vi "NewProjectDialog.vi"(10 "Project XML":string="<ProjectTemplate>\n  <Title localize=\"yes\">队列状态机</Title>\n  <Description localize=\"yes\">本模板可用于创建事件驱动的用户界面状态机。</Description>\n  <Filter localize=\"yes\">桌面：模板</Filter>\n  <Keywords localize=\"yes\">状态;状态机;队列;事件;处理器;消息</Keywords>\n  <LocationPath>Core/Queued State Machine</LocationPath>\n  <ProjectPath>Queued State Machine.lvproj</ProjectPath>\n  <ListboxImagePath>images/qsm_small.png</ListboxImagePath>\n  <GalleryImagePaths>images/qsm.png;images/knob.jpg</GalleryImagePaths>\n  <DocumentationPath>html/Project Documentation.html</DocumentationPath>\n  <CustomVIMode>None</CustomVIMode>\n  <CustomVIPath></CustomVIPath>\n</ProjectTemplate>" caption="项目XML", 11 "Calling Mode":T1 caption="调用模式") -> ()   [LabVIEW 2016]
uses:
  <resource>/dialog/NewProjectWizard/NewProjectDialogCallingModes.ctl
  <resource>/dialog/NewProjectWizard/MetaDataObj/MetaDataObj.lvclass
  <resource>/dialog/NewProjectWizard/SpecPage/Base/BaseSpecPage.lvclass
  <resource>/dialog/NewProjectWizard/Operation to Log.ctl
  <vilib>/event_ctls.llb/eventvkey.ctl
  <resource>/dialog/NewProjectWizard/MetaDataObj/MetaDataObj.lvclass/MetaDataObj.ctl
  <resource>/dialog/NewProjectWizard/Spec Page Interface.ctl
  <resource>/dialog/NewProjectWizard/MetaDataObj/Accessors/Write Project Root.vi
  <resource>/dialog/NewProjectWizard/MetaDataObj/Accessors/Read Project Root.vi
  <resource>/dialog/NewProjectWizard/MetaDataObj/Accessors/Read File Prefix.vi
  <resource>/dialog/NewProjectWizard/MetaDataObj/Accessors/Read Project Name.vi
  <resource>/dialog/NewProjectWizard/MetaDataObj/Accessors/Read Overlay Pixmap.vi
  <resource>/dialog/NewProjectWizard/MetaDataObj/Accessors/Read Custom VI Mode.vi
  <resource>/dialog/NewProjectWizard/MetaDataObj/Accessors/Read Custom VI Path.vi
  <resource>/dialog/NewProjectWizard/MetaDataObj/Accessors/Read Title.vi
  <resource>/dialog/NewProjectWizard/MetaDataObj/Accessors/Read Project Path.vi
  <vilib>/LabVIEW Icon API/lv_icon/Classes/Icon/Icon.lvclass
  <helpdir>/_LaunchHelp.vi
  <resource>/dialog/NewProjectWizard/Init Search Page.vi
  <resource>/dialog/NewProjectWizard/Build Error String.vi
  <resource>/dialog/NewProjectWizard/Log Project Selection.vi
  <resource>/dialog/NewProjectWizard/Process Tab Key.vi
  <resource>/dialog/lvconfig.llb/LV Config Read Pathlist.vi
  <resource>/dialog/NewProjectWizard/MetaDataObj/Convert To Child Class.vi
  <resource>/dialog/NewProjectWizard/Init Spec Page.vi
  <resource>/dialog/NewProjectWizard/Defer Panel Updates.vi
  <resource>/dialog/NewProjectWizard/ValidateFilePath.vi
  <resource>/dialog/lvconfig.llb/LV Config Write Pathlist.vi
  <resource>/dialog/NewProjectWizard/Project Copying/CreateUserProject.vi
  <resource>/dialog/NewProjectWizard/Project Copying/NI_NPW_Project Copying.lvlib
  <vilib>/Utility/cursorutil.llb/Set Busy.vi
  <resource>/dialog/NewProjectWizard/Project Copying/SaveTemplatePathToINI.vi
  <resource>/dialog/NewProjectWizard/FindRecentItem.vi
  <resource>/dialog/NewProjectWizard/Loading Project Info/LoadTemplateFromXML.vi
  <resource>/dialog/NewProjectWizard/Loading Project Info/NI_NPW_Loading Project Info.lvlib
panel:
  in  "Dummy Template":refnum<class "MetaDataObj.lvclass"> caption="虚设模板"
  in  "recent_item":path caption="最近项"
  out "Title":string="消息:" caption="标题"
  in  "Spec Page Title":string="配置新项目：%s" caption="规范页标题"
  in  "Search Page Title":string="选择项目起始位置：" caption="搜索页标题"
  out "Error Messages":string caption="错误信息"
  out "CurPage Ctrl #n":refnum<vi> caption="当前页Ctrl #n"
  out "CurPage Ctrl #1":refnum<vi> caption="当前页Ctrl #1"
  out "Search Page":refnum<vi> caption="搜索页"
  out "SpecPage Ctrl #n":refnum<vi> caption="规范页Ctrl #n"
  out "SearchPage Ctrl #n":refnum<vi> caption="搜索页Ctrl #n"
  out "SpecPage Ctrl #1":refnum<vi> caption="规范页Ctrl #1"
  out "SearchPage Ctrl #1":refnum<vi> caption="搜索页Ctrl #1"
  in  "Finish":string="完成" caption="完成"
  in  "Next":string="下一步" caption="下一步"
  in  "Help":bool caption="帮助"
  in  "Cancel":bool caption="取消"
  in  "Next":bool caption="下一步"
  in  "Back":bool caption="上一步"
  in  "File Not Found":string="LabVIEW无法找到项目的源文件。" caption="未找到文件"
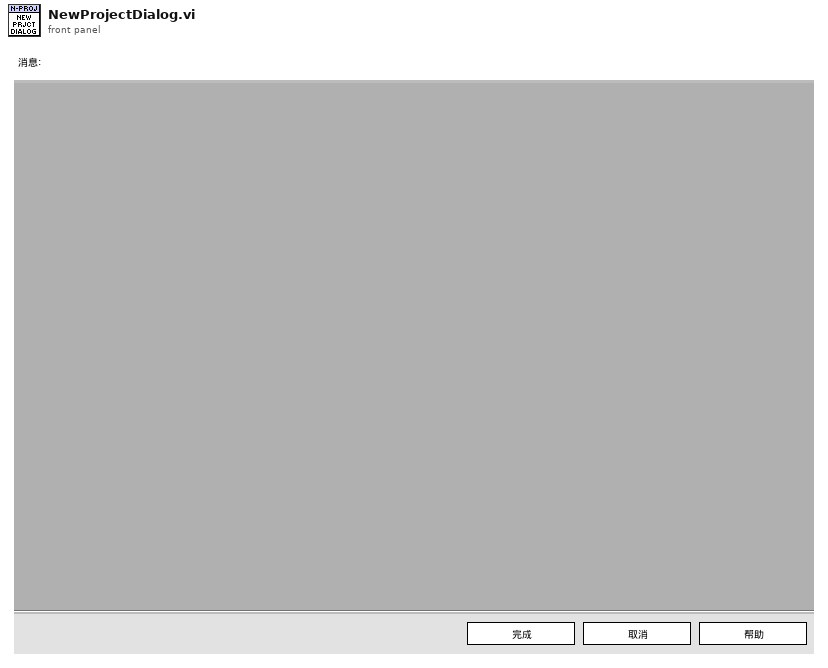
[diagram p1: front panel]
types:
  T1 = typedef "NewProjectDialogCallingModes.ctl" = enum16{"Default", "Open to 2nd Page", "Open Recent Item"}
  T2 = enum32{"Invalid", "Standard", "Closed", "Hidden", "Minimized", "Maximized"}
  T3 = enum8{"Enabled", "Disabled", "Disabled and Grayed Out"}
  T4 = typedef "CustomVIModes.ctl" = enum16{"None", "AfterPage1", "AfterPage2WithUI", "AfterPage2NoUI"}
  T5 = typedef "Operation to Log.ctl" = enum16{"Create", "Cancel", "MoreInfoLink"}
  T6 = typedef "eventvkey.ctl" = enum16{"ASCII", "Enter", "Return", "Shift", "Ctrl", "Alt", "Cmd", "Opt", "Caps", "NumLock", "Clear", "Break", "Up", "Down", "Left", "Right", "Insert", "Delete", "Home", "End", "PageUp", "PageDown", "Escape", "Help", "Pause", "ScrollLock", "F1", "F2", "F3", "F4", "F5", "F6", "F7", "F8", "F9", "F10", "F11", "F12", "F13", "F14", "F15", "F16", "F17", "F18", "F19", "F20", "F21", "F22", "F23", "F24", "Play", "VolumeUp", "VolumeDown", "Mute", "Two Byte Char"}
  T7 = typedef "Spec Page Interface.ctl" = cluster{"\"Tab Forward To\" Refnum":refnum<vi>, "\"Tab Backward To\" Refnum":refnum<vi>, "Errors":refnum<user-event>, "Quit":refnum<user-event>}
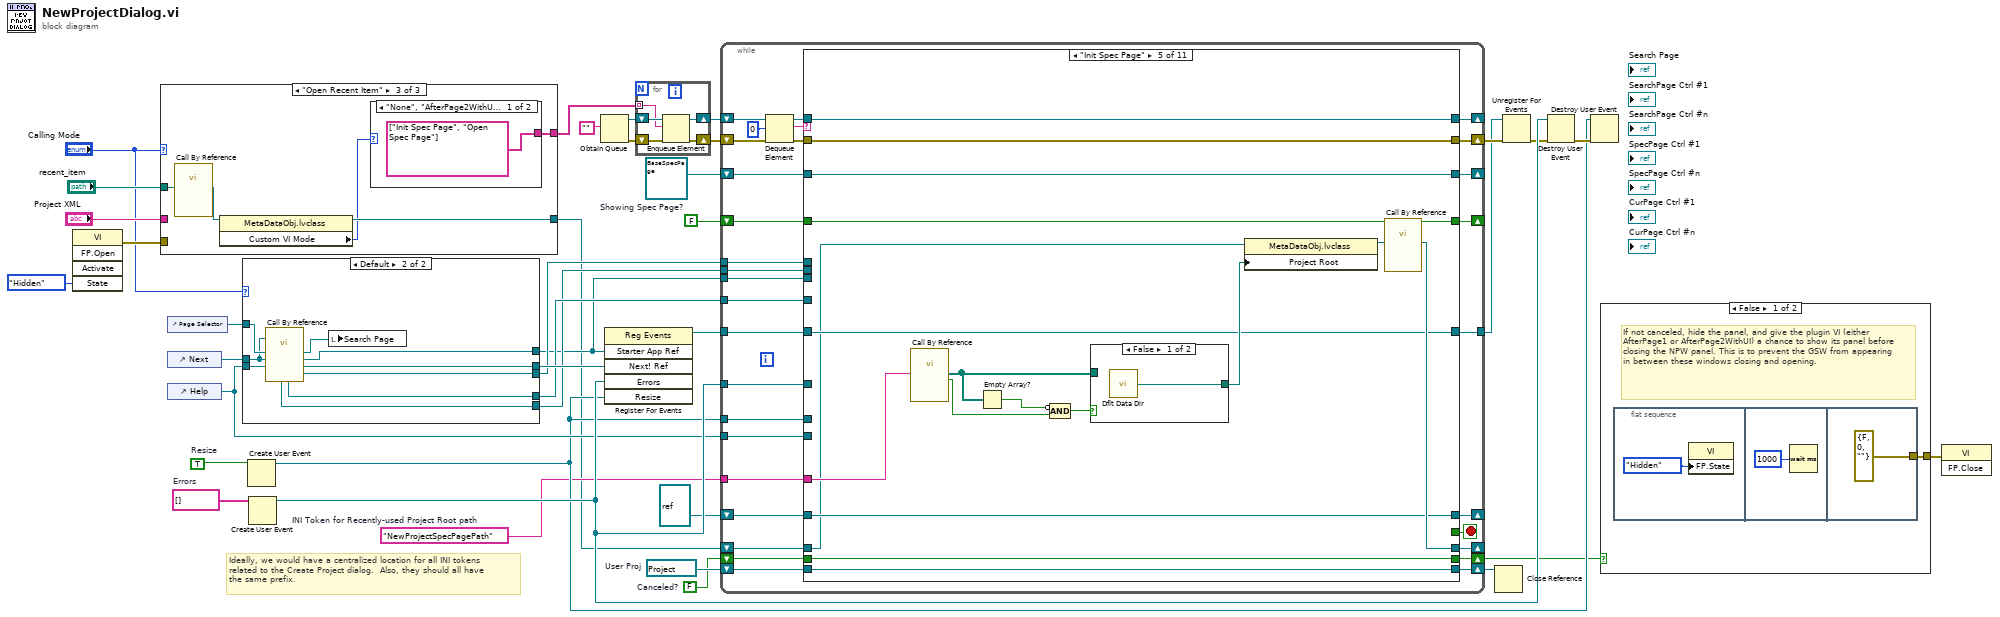
[diagram p0: block diagram]
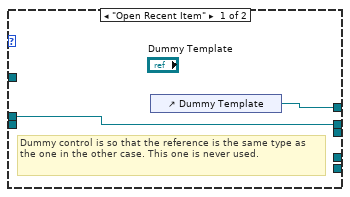
[diagram p3: hidden frame]
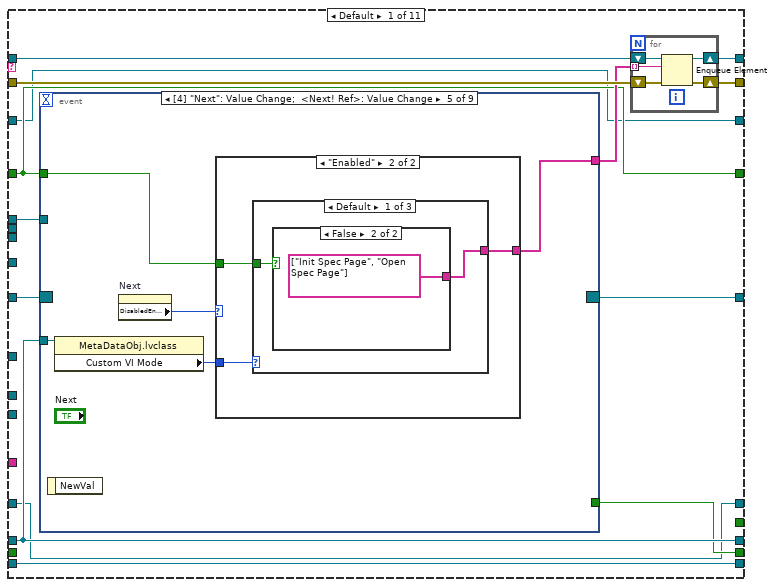
[diagram p4: hidden frame]
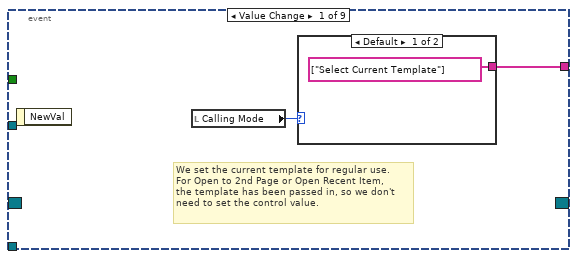
[diagram p5: hidden frame]
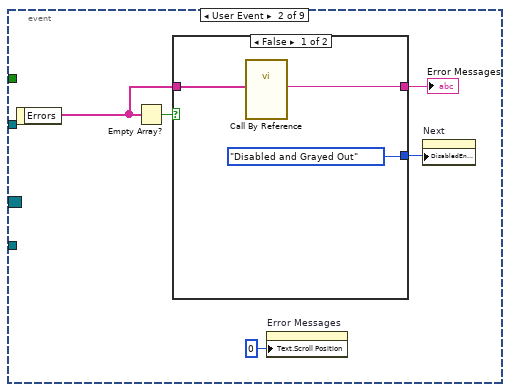
[diagram p7: hidden frame]
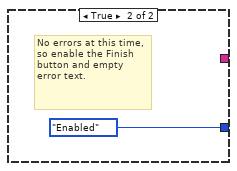
[diagram p8: hidden frame]
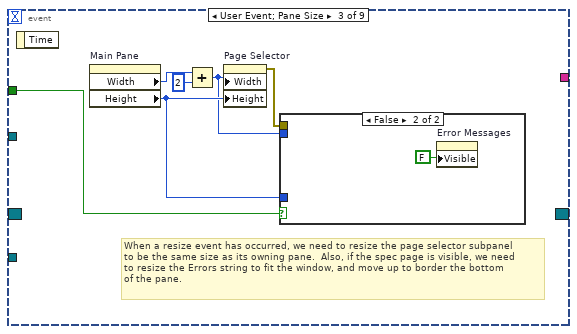
[diagram p9: hidden frame]
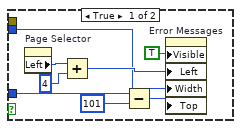
[diagram p10: hidden frame]
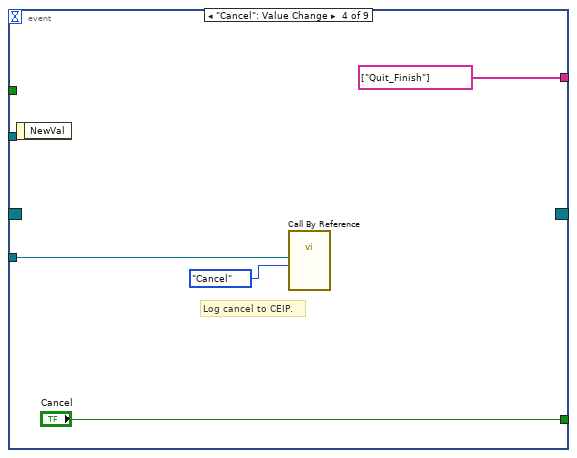
[diagram p11: hidden frame]
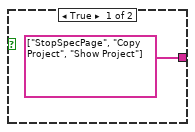
[diagram p13: hidden frame]
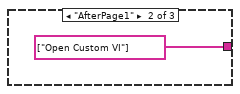
[diagram p14: hidden frame]
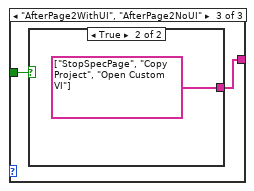
[diagram p15: hidden frame]
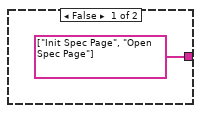
[diagram p16: hidden frame]
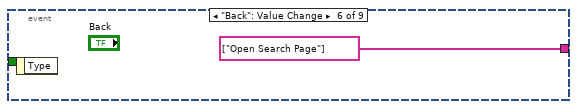
[diagram p17: hidden frame]
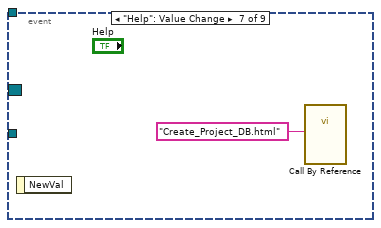
[diagram p18: hidden frame]
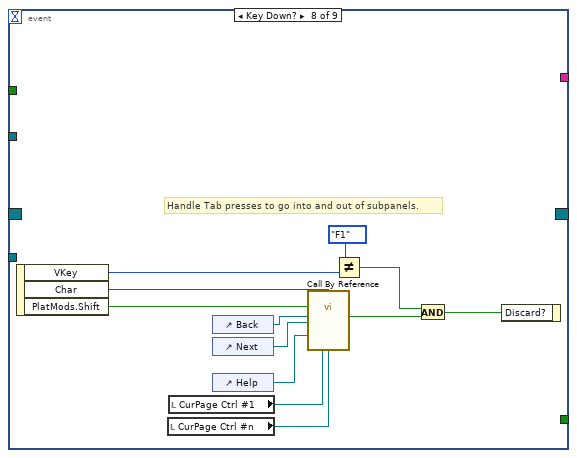
[diagram p19: hidden frame]
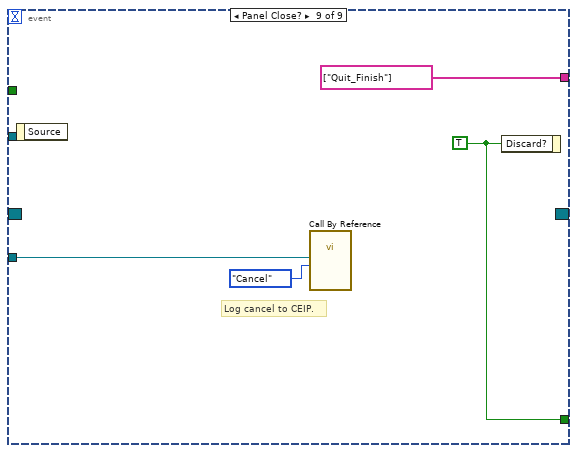
[diagram p20: hidden frame]
diagram:
  w10 = FALSE  # Canceled?
  w12 = "NewProjectSpecPagePath"  # INI Token for Recently-used Project Root path
  w18 = refnum<vi> refnum  # User Proj
  w19 = FALSE  # Showing Spec Page?
  w28 = TRUE  # Resize
  w29 = string[] []  # Errors
  # "Ideally, we would have a centralized location for all INI tokens\nrelated to the Create Project dialog.  Also, they should all have\nthe same prefix."
  n1 = invoke class="VI" method="FP.Open"("State"=T2."Hidden") -> (error out=w17:errorcluster)  [unwired: 4 in, 4 out]
  n2 = case shown="\"Open Recent Item\"" "Calling Mode" {
    tunnel: [string[] ["Select Current Template", "Open Search Page"] ("Initial States") string[] ["Init Spec Page", "Open Spec Page"] ("Initial States") w48] -> w38
    tunnel: "Project XML" -> [_ w41 _]
    tunnel: [_ w40 w47] -> w3
    tunnel: "recent_item" -> [_ _ w45]
    tunnel: w17 -> [_ _ _]
    frame Default {
    }
    frame "Open to 2nd Page" {
      # "(In this mode, the user passes\nin XML for the template that\nthey want.)"
      n3 = call-by-ref "?"("XML String In"=w41) -> ("Template Out"=w40:refnum<class "MetaDataObj.lvclass">)  [unwired: 11 in, 3 out]
      n4 = property on="Back" class="Bool"("DisabledEnum"=T3."Disabled and Grayed Out" ("Disabled")) -> ()  [unwired: 2 in, 2 out]
    }
    frame "Open Recent Item" {
      n5 = call-by-ref "?"("recent_item"=w45) -> ("MetaDataObj out"=w44:refnum<class "MetaDataObj.lvclass">)  [unwired: 11 in, 3 out]
      n6 = property class="MetaDataObj.lvclass"(reference=w44) -> (reference out=w47:refnum<class "MetaDataObj.lvclass">, "Custom VI Mode"=w46:T4)  [unwired: 1 in, 1 out]
      n7 = case shown="\"None\", \"AfterPage2WithUI\", \"AfterPage2NoUI\"" w46 {
        tunnel: [string[] ["Init Spec Page", "Open Spec Page"] ("Initial States") string[] ["Open Custom VI"] ("Initial States")] -> w48
        frame "None", "AfterPage2WithUI", "AfterPage2NoUI" {
        }
        frame "AfterPage1" {
        }
      }
    }
  }
  n8 = control-ref of="Page Selector"() -> (w30:refnum<vi>)
  n9 = control-ref of="Next"() -> (w15:refnum<vi>)
  n10 = control-ref of="Help"() -> (w16:refnum<vi>)
  n11 = case shown="Default" "Calling Mode" {
    tunnel: [w51 w53] -> w7
    tunnel: [w52 w61] -> w37
    tunnel: [_ w60] -> w34
    tunnel: [_ w59] -> w33
    tunnel: w30 -> [_ w57]
    tunnel: w16 -> [_ w56]
    tunnel: w15 -> [w52 w54]
    tunnel: [_ w55] -> w13
    frame "Open Recent Item" {
      # "Dummy control is so that the reference is the same type as the one in the other case. This one is never used."
      n12 = control-ref of="Dummy Template"() -> (w51:refnum<vi>)
    }
    frame Default {
      n13 = call-by-ref "?"("Next Button"=w54, "\"Tab Backward To\" Refnum"=w56, "\"Tab Forward To\" Refnum"=w54, "SubPanel"=w57) -> ("Additional Search Ref"=w55:refnum<vi>, "Next! Ref"=w61:refnum<vi>, "Starter App Ref"=w53:refnum<vi>, "Search Page Ref"=w58:refnum<vi>, "SearchPage Ctrl #n Ref"=w60:refnum<vi>, "SearchPage Ctrl #1 Ref"=w59:refnum<vi>)  [unwired: 4 in, 2 out]
      n14 = local write "Search Page"(w58) -> ()
    }
  }
  n15 = Create User Event(user event datatype=w28) -> (user event=w14:refnum<user-event>)  [unwired: 1 in, 1 out]
  n16 = Create User Event(user event datatype=w29) -> (user event=w35:refnum<user-event>)  [unwired: 1 in, 1 out]
  n17 = Obtain Queue(element data type="") -> (queue out=w23:refnum<queue>, error out=w22:errorcluster)  [unwired: 4 in, 1 out]
  n18 = register-events(w7, w37, w35, w14) -> (reference out=w24:refnum<event-registration>)  [unwired: 2 in, 1 out]
  n19 = for {
    shift-right: [w66] -> w26
    shift-left: w23 -> [w64]
    shift-right: [w65] -> w25
    shift-left: w22 -> [w63]
    tunnel: w38 -> [w62] mode=indexing
    n20 = Enqueue Element(queue=w64, element=w62, error in (no error)=w63) -> (queue out=w66:refnum<queue>, error out=w65:errorcluster)  [unwired: 1 in, 1 out]
  }
  n21 = while {
    shift-right: [w91] -> _
    shift-left: w26 -> [w96]
    shift-right: [w90] -> w21
    shift-left: w25 -> [w95]
    shift-right: [w86] -> _
    shift-left: w3 -> [w87]
    tunnel: w7 -> [w85]
    tunnel: w35 -> [w84]
    tunnel: w34 -> [w83]
    tunnel: w33 -> [w82]
    tunnel: w14 -> [w81]
    shift-right: [w79] -> _
    shift-left: w19 -> [w80]
    shift-right: [w77] -> w11
    shift-left: w18 -> [w78]
    tunnel: w16 -> [w76]
    tunnel: w13 -> [w75]
    tunnel: w12 -> [w74]
    shift-right: [w72] -> w2
    shift-left: w10 -> [w73]
    shift-right: [w71] -> _
    shift-left: refnum<vi> refnum ("vi reference") -> [w70]
    tunnel: w24 -> [w89]
    tunnel: [w69] -> w8
    shift-right: [w68] -> _
    shift-left: refnum<class "BaseSpecPage.lvclass"> refnum ("BaseSpecPage out") -> [w67]
    stop <- w88 stop-if-true
    n22 = Dequeue Element(queue=w96, timeout in ms (-1)=0, error in (no error)=w95) -> (queue out=w94:refnum<queue>, element=w92:string, error out=w93:errorcluster)  [unwired: 1 out]
    n23 = case shown="\"Init Spec Page\"" w92 {
      tunnel: w94 -> [w108 w193 w214 w252 w299 w306 w373 w404 w460 w475 w500]
      tunnel: w93 -> [w109 w192 w210 w249 w298 w305 w378 w405 w459 w473 w499]
      tunnel: [w111 w193 w214 w251 w299 w306 w372 w403 w458 w474 w500] -> w91
      tunnel: [w110 w192 w210 w250 w298 w305 w376 w402 w457 w472 w499] -> w90
      tunnel: w89 -> [w107 w188 w199 w245 w294 w304 w385 w410 w455 w477 w489]
      tunnel: [_ _ _ _ _ _ _ _ _ _ TRUE] -> w88
      tunnel: w87 -> [w105 _ w213 w246 w283 w323 w374 w416 w461 w469 w486]
      tunnel: [w105 w190 w213 w246 w295 w323 w386 w416 w461 w469 w486] -> w86
      tunnel: w85 -> [_ w189 _ _ _ _ _ _ _ _ _]
      tunnel: w84 -> [_ _ _ _ _ w322 _ _ _ _ _]
      tunnel: w83 -> [_ _ w212 _ _ _ _ _ _ _ _]
      tunnel: w82 -> [_ _ w211 _ _ _ _ _ _ _ _]
      tunnel: [w104 w188 w199 w245 w294 w304 w385 w410 w455 w477 w489] -> w69
      tunnel: w81 -> [_ _ w202 _ _ w319 _ _ _ _ _]
      tunnel: w80 -> [w103 w187 _ w244 w293 _ w371 w409 w454 w476 w488]
      tunnel: [w103 w187 w207 w244 w293 w318 w371 w409 w454 w476 w488] -> w79
      tunnel: w78 -> [w102 w186 w205 w242 w288 w317 w384 w408 w453 w470 w487]
      tunnel: [w102 w186 w205 w242 w288 w317 w384 w407 refnum<vi> refnum ("User Proj") w470 w487] -> w77
      tunnel: w76 -> [_ _ _ _ _ w315 _ _ _ _ _]
      tunnel: w75 -> [w101 _ _ _ _ _ _ _ _ _ _]
      tunnel: w74 -> [_ _ _ _ w287 _ _ w406 _ _ _]
      tunnel: w73 -> [_ w185 w198 w241 w286 w312 w383 w401 w450 w467 w485]
      tunnel: [w100 w185 w198 w241 w286 w312 w383 w401 w450 w467 w485] -> w72
      tunnel: [w99 w184 w197 w240 w285 w311 w382 w400 w449 w466 w484] -> w71
      tunnel: w70 -> [w99 w184 w197 w239 w285 w311 w382 w400 w449 w466 w484]
      tunnel: [w98 w183 w196 w238 w284 w310 w381 w399 w448 w465 w478] -> w68
      tunnel: w67 -> [w98 w183 w196 w238 w284 w308 w380 w399 w448 w465 w478]
      frame Default {
        n24 = event shown="[4] \"Next\": Value Change;  <Next! Ref>: Value Change" {
          selector: w107 -> [_ _ _ _ _ _ _ _ _]
          dyn-events: [_ _ _ _ _ _ _ _ _] -> w104
          timeout: _ -> [_ _ _ _ _ _ _ _ _]
          tunnel: [w118 _ _ string[] ["Quit_Finish"] w151 string[] ["Open Search Page"] _ _ string[] ["Quit_Finish"]] -> w106
          tunnel: w105 -> [_ _ _ w146 w150 _ _ _ w181]
          tunnel: w103 -> [_ _ w134 _ w149 _ _ _ _]
          tunnel: w101 -> [_ _ _ _ _ _ _ _ _]
          tunnel: [_ _ _ "Cancel" _ _ _ _ w179] -> w100
          event Value Change {
            # "We set the current template for regular use.\nFor Open to 2nd Page or Open Recent Item,\nthe template has been passed in, so we don't\nneed to set the control value."
            n25 = event-data() -> ()  [unwired: 1 in, 1 out]
            n26 = local read "Calling Mode"() -> (w117:T1)
            n27 = case shown="Default" w117 {
              tunnel: [string[] ["Select Current Template"] _] -> w118
              frame Default {
              }
              frame "Open to 2nd Page", "Open Recent Item" {
              }
            }
          }
          event User Event {
            n28 = event-data() -> ("Errors"=w123:string[])  [unwired: 1 in]
            n29 = Empty Array?(array=w123) -> (empty?=w124:bool)
            n30 = case shown="False" w124 {
              tunnel: w123 -> [w125 _]
              tunnel: [T3."Disabled and Grayed Out" ("Disabled") T3."Enabled" ("Disabled")] -> w120
              tunnel: [w126 _] -> w122
              frame False {
                n31 = call-by-ref "?"("Errors"=w125) -> ("String"=w126:string)  [unwired: 12 in, 2 out]
              }
              frame True {
                # "No errors at this time, so enable the Finish button and empty error text."
              }
            }
            "Error Messages" <- w122
            n32 = property on="Error Messages" class="Str"("Text.Scroll Position"=u32 0) -> ()  [unwired: 2 in, 2 out]
            n33 = property on="Next" class="Bool"("DisabledEnum"=w120) -> ()  [unwired: 2 in, 2 out]
          }
          event User Event; Pane Size {
            # "When a resize event has occurred, we need to resize the page selector subpanel\nto be the same size as its owning pane.  Also, if the spec page is visible, we need\nto resize the Errors string to fit the window, and move up to border the bottom\nof the pane."
            n34 = event-data() -> ()  [unwired: 1 in, 1 out]
            n35 = property on="Main Pane" class="Pane"() -> ("Width"=w131:u32, "Height"=w130:u32)  [unwired: 2 in, 2 out]
            n36 = Add(x=w131, y=u32 2 ("x")) -> (x+y=w129:u32)
            n37 = property on="Page Selector" class="SubPnl"("Width"=w129, "Height"=w130) -> (error out=w133:errorcluster)  [unwired: 2 in, 1 out]
            n38 = case shown="False" w134 {
              tunnel: w129 -> [w138 _]
              tunnel: w133 -> [_ _]
              tunnel: w130 -> [w137 _]
              frame True {
                n39 = property on="Page Selector" class="SubPnl"() -> ("Left"=w141:i32)  [unwired: 2 in, 2 out]
                n40 = Add(x=w141, y=4 ("x")) -> (x+y=w140:i32)
                n41 = Subtract(x=w137, y=u32 101) -> (x-y=w136:u32)
                n42 = property on="Error Messages" class="Str"("Visible"=TRUE, "Left"=w140, "Width"=w138, "Top"=w136) -> ()  [unwired: 2 in, 2 out]
              }
              frame False {
                n43 = property on="Error Messages" class="Str"("Visible"=FALSE) -> ()  [unwired: 2 in, 2 out]
              }
            }
          }
          event "Cancel": Value Change {
            # "Log cancel to CEIP."
            n44 = event-data() -> ()  [unwired: 1 in, 1 out]
            n45 = call-by-ref "?"("Operation to Log"=Operation_to_Log."Cancel", "MetaDataObj in"=w146) -> ()  [unwired: 12 in, 2 out]
          }
          event "Next": Value Change {
            n46 = event-data() -> ()  [unwired: 1 in, 1 out]
            n47 = property class="MetaDataObj.lvclass"(reference=w150) -> ("Custom VI Mode"=w152:T4)  [unwired: 1 in, 2 out]
            n48 = property on="Next" class="Bool"() -> ("DisabledEnum"=w148:T3)  [unwired: 2 in, 2 out]
            n49 = case shown="\"Enabled\"" w148 {
              tunnel: w152 -> [_ w155]
              tunnel: [_ w154] -> w151
              tunnel: w149 -> [_ w153]
              frame Default {
                # "If Next is disabled, don't allow anything to advance to the next page"
              }
              frame "Enabled" {
                n50 = case shown="Default" w155 {
                  tunnel: [w157 string[] ["Open Custom VI"] w161] -> w154
                  tunnel: w153 -> [w156 _ w162]
                  frame Default {
                    n51 = case shown="False" w156 {
                      tunnel: [string[] ["StopSpecPage", "Copy Project", "Show Project"] string[] ["Init Spec Page", "Open Spec Page"]] -> w157
                      frame True {
                      }
                      frame False {
                      }
                    }
                  }
                  frame "AfterPage1" {
                  }
                  frame "AfterPage2WithUI", "AfterPage2NoUI" {
                    n52 = case shown="True" w162 {
                      tunnel: [string[] ["Init Spec Page", "Open Spec Page"] string[] ["StopSpecPage", "Copy Project", "Open Custom VI"]] -> w161
                      frame False {
                      }
                      frame True {
                      }
                    }
                  }
                }
              }
            }
          }
          event "Back": Value Change {
            n53 = event-data() -> ()  [unwired: 1 in, 1 out]
          }
          event "Help": Value Change {
            n54 = event-data() -> ()  [unwired: 1 in, 1 out]
            n55 = call-by-ref "?"("HTML filename"="Create_Project_DB.html") -> ()  [unwired: 8 in, 3 out]
          }
          event Key Down? {
            # "Handle Tab presses to go into and out of subpanels."
            n56 = event-data() -> ("VKey"=w170:T6, "Char"=w177:i16, "PlatMods.Shift"=w176:bool)  [unwired: 1 in]
            n57 = local read "CurPage Ctrl #n"() -> (w174:refnum<vi>)
            n58 = local read "CurPage Ctrl #1"() -> (w175:refnum<vi>)
            n59 = control-ref of="Back"() -> (w173:refnum<vi>)
            n60 = control-ref of="Next"() -> (w172:refnum<vi>)
            n61 = control-ref of="Help"() -> (w171:refnum<vi>)
            n62 = call-by-ref "?"("Back"=w173, "Shift"=w176, "Char"=w177, "Next"=w172, "Help"=w171, "CurPage Ctrl #1"=w175, "CurPage Ctrl #n"=w174) -> ("Discard Key Down Event?"=w178:bool)  [unwired: 10 in, 2 out]
            n63 = Not Equal?(x=eventvkey."F1", y=w170) -> (x != y?=w167:bool)
            n64 = And(x=w167, y=w178) -> (x .and. y?=w168:bool)
            n65 = event-data("Discard?"=w168) -> ()  [unwired: 1 in, 1 out]
          }
          event Panel Close? {
            w179 = TRUE ("Discard?")
            # "Log cancel to CEIP."
            n66 = event-data() -> ()  [unwired: 1 in, 1 out]
            n67 = call-by-ref "?"("Operation to Log"=Operation_to_Log."Cancel", "MetaDataObj in"=w181) -> ()  [unwired: 12 in, 2 out]
            n68 = event-data("Discard?"=w179) -> ()  [unwired: 1 in, 1 out]
          }
        }
        n69 = for {
          tunnel: w106 -> [w112] mode=indexing
          shift-right: [w116] -> w111
          shift-left: w108 -> [w113]
          shift-right: [w115] -> w110
          shift-left: w109 -> [w114]
          n70 = Enqueue Element(queue=w113, element=w112, error in (no error)=w114) -> (queue out=w116:refnum<queue>, error out=w115:errorcluster)  [unwired: 1 in, 1 out]
        }
      }
      frame "Select Current Template" {
        w194 = refnum<class "MetaDataObj.lvclass"> refnum  # Dummy Template
        n71 = property class="Ctl"(reference=w189) -> (error out=w191:errorcluster, "Value"=w195:variant)  [unwired: 1 in, 1 out]
        n72 = Variant To Data(error in=w191, type=w194, Variant=w195) -> (data=w190:refnum<class "MetaDataObj.lvclass">)  [unwired: 1 out]
      }
      frame "Open Search Page" {
        n73 = flat-sequence {
          tunnel: w211 -> [w217]
          tunnel: w212 -> [w218]
          tunnel: [w218] -> w209
          tunnel: [w217] -> w208
          tunnel: [w216] -> w203
          tunnel: w202 -> [w216]
          tunnel: [w215] -> w200
          tunnel: w209 -> [w226]
          tunnel: w208 -> [w225]
          tunnel: [w222] -> w206
          tunnel: [w220] -> w204
          tunnel: w203 -> [w220]
          tunnel: [w219] -> w201
          tunnel: w200 -> [w219]
          tunnel: [w237] -> w207
          tunnel: w206 -> [w237]
          tunnel: w204 -> [w236]
          tunnel: w201 -> [w235]
          frame #0 {
            n74 = property class="VI"() -> ("FP.State"=w215:T2)  [unwired: 2 in, 2 out]
          }
          frame #1 {
            w222 = FALSE  # Showing Spec Page?
            n75 = local write "CurPage Ctrl #1"(w225) -> ()
            n76 = local write "CurPage Ctrl #n"(w226) -> ()
            n77 = property on="Error Messages" class="Str"("Visible"=FALSE) -> ()  [unwired: 2 in, 2 out]
            n78 = local read "Search Page"() -> (w227:refnum<vi>)
            n79 = property on="Back" class="Bool"("Visible"=FALSE) -> ()  [unwired: 2 in, 2 out]
            n80 = invoke on="Page Selector" class="SubPnl" method="Insert VI"("VI Ref"=w227) -> ()  [unwired: 3 in, 4 out]
            "Title" <- "Search Page Title"
          }
          frame #2 {
            w233 = T2."Maximized" ("x")
            # "Fire resize event once\nSearch Page is visible"
            n81 = Equal?(x=w233, y=w235) -> (x = y?=w234:bool)
            n82 = Generate User Event(user event=w236, event data cluster=TRUE ("event data")) -> ()  [unwired: 2 in, 2 out]
            n83 = Select(t=w233, s=w234, f=T2."Standard" ("Front Panel Window:State")) -> (s? t:f=w231:T2)
            n84 = property on="Next" class="Bool"("BoolText.Text"="Next", "DisabledEnum"=T3."Enabled" ("Disabled")) -> ()  [unwired: 2 in, 2 out]
            n85 = property class="VI"("FP.State"=w231) -> ()  [unwired: 2 in, 2 out]
          }
        }
      }
      frame "Open Custom VI" {
        n86 = property class="MetaDataObj.lvclass"(reference=w246) -> (reference out=w243:refnum<class "MetaDataObj.lvclass">, error out=w253:errorcluster, "Custom VI Mode"=w247:T4, "Custom VI Path"=w254:path)  [unwired: 1 in]
        n87 = case shown="\"AfterPage2WithUI\"" w247 {
          tunnel: w254 -> [_ w262 w270 w282]
          tunnel: w253 -> [_ w259 w269 w281]
          tunnel: w243 -> [_ _ w264 w277]
          tunnel: w242 -> [_ _ _ w272]
          tunnel: [w255 w256 w263 w271] -> w240
          tunnel: w239 -> [w255 _ _ w271]
          frame Default {
          }
          frame "AfterPage1" {
            # "Auto dispose ref so the plugin does not get cleaned up when this VI goes idle."
            n88 = Open VI Reference(vi path=w262, error in (no error)=w259) -> (vi reference=w261:refnum<vi>, error out=w258:errorcluster)  [unwired: 4 in]
            n89 = invoke class="VI" method="Run VI"(reference=w261, error in=w258, "Wait until done"=FALSE ("Wait Until Done"), "Auto Dispose Ref"=TRUE ("Auto Dispose Reference")) -> (reference out=w256:refnum<vi>)  [unwired: 1 in, 4 out]
          }
          frame "AfterPage2WithUI" {
            w265 = 128  # fire and forget
            n90 = Open VI Reference(type specifier VI Refnum (for type only)=refnum<vi> refnum, vi path=w270, options=w265, error in (no error)=w269) -> (vi reference=w268:refnum<vi>, error out=w266:errorcluster)  [unwired: 2 in]
            n91 = call-by-ref "Start Asynchronous Call"(reference=w268, error in=w266, "MetaDataObj"=w264) -> (reference out=w263:refnum<vi>)  [unwired: 11 in, 1 out]
          }
          frame "AfterPage2NoUI" {
            # "Just in case the custom scripting did not close the progress bar, make sure it gets closed"
            n92 = Open VI Reference(type specifier VI Refnum (for type only)=refnum<vi> refnum, vi path=w282, error in (no error)=w281) -> (vi reference=w280:refnum<vi>, error out=w278:errorcluster)  [unwired: 3 in]
            n93 = call-by-ref "?"(reference=w280, error in=w278, "DNL_MetaDataObj"=w277, "Project"=w272) -> (reference out=w276:refnum<vi>, error out=w275:errorcluster)  [unwired: 10 in]
            n94 = Close Reference(reference=w276, error in (no error)=w275) -> (error out=w274:errorcluster)
            n95 = call <vilib>:"Clear Errors.vi"("error in (no error)"=w274) -> ("error out"=w273:errorcluster)  [unwired: 5 in, 1 out]
            n96 = call <resource>:"Close Create Project Progress Bar.vi"("error in (no error)"=w273, "Project"=w272) -> ()  [unwired: 8 in, 2 out]
          }
        }
        n97 = Enqueue Element(queue=w252, element="Quit", error in (no error)=w249) -> (queue out=w251:refnum<queue>, error out=w250:errorcluster)  [unwired: 1 in, 1 out]
      }
      frame "Init Spec Page" {
        n98 = call-by-ref "?"("key"=w287) -> ("found?"=w292:bool, "value"=w290:path[])  [unwired: 6 in, 3 out]
        n99 = Empty Array?(array=w290) -> (empty?=w289:bool)
        n100 = Compound Arithmetic op=AND(invert w289, w292) -> (w291:bool)
        n101 = case shown="False" w291 {
          tunnel: w290 -> [_ w303]
          tunnel: [w300 w301] -> w297
          frame False {
            n102 = call <vilib>:"Dflt Data Dir.vi"() -> ("App:Default Data Directory"=w300:path)
          }
          frame True {
            n103 = Index Array(array=w303) -> (element=w302:path)  [unwired: 1 in]
            n104 = Strip Path(path=w302) -> (stripped path=w301:path)  [unwired: 1 out]
          }
        }
        n105 = property class="MetaDataObj.lvclass"(reference=w283, "Project Root"=w297) -> (reference out=w296:refnum<class "MetaDataObj.lvclass">)  [unwired: 1 in, 1 out]
        n106 = call-by-ref "?"("MetaDataObj in"=w296) -> ("MetaDataObj out"=w295:refnum<class "MetaDataObj.lvclass">)  [unwired: 12 in, 2 out]
      }
      frame "Open Spec Page" {
        n107 = flat-sequence {
          tunnel: w322 -> [w330]
          tunnel: [w330] -> w321
          tunnel: [w327] -> w320
          tunnel: w319 -> [w327]
          tunnel: [w326] -> w316
          tunnel: w315 -> [w326]
          tunnel: [w325] -> w313
          tunnel: w308 -> [w324]
          tunnel: [w324] -> w307
          tunnel: w323 -> [w332]
          tunnel: w321 -> [w354]
          tunnel: w320 -> [w351]
          tunnel: w316 -> [w350]
          tunnel: [w345] -> w314
          tunnel: w313 -> [w344]
          tunnel: [w340] -> w309
          tunnel: w307 -> [w337]
          tunnel: [TRUE ("Showing Spec Page?")] -> w318
          tunnel: w314 -> [w368]
          tunnel: [w367] -> w310
          tunnel: w309 -> [w367]
          frame #0 {
            n108 = control-ref of="This VI"() -> (w328:refnum<vi>)
            n109 = property class="VI"() -> ("FP.State"=w325:T2)  [unwired: 2 in, 2 out]
            n110 = call-by-ref "?"("Defer?"=TRUE ("Visible"), "VI in"=w328) -> ()  [unwired: 11 in, 3 out]
          }
          frame #1 {
            w336 = refnum<user-event> refnum  # Null Event
            w347 = T2."Maximized" ("x")
            w355 = T7 {"\"Tab Forward To\" Refnum"=refnum, "\"Tab Backward To\" Refnum"=refnum, "Errors"=refnum, "Quit"=refnum}  # Wizard Interface
            # "Calling close makes debugging easier if we can have panel open initially."
            # "Fire stop event in case a spec page is already running."
            n111 = property class="MetaDataObj.lvclass"(reference=w332) -> ("Title"=w331:string)  [unwired: 1 in, 2 out]
            n112 = property on="Next" class="Bool"("BoolText.Text"="Finish") -> ()  [unwired: 2 in, 2 out]
            n113 = Generate User Event(user event=w351, event data cluster=TRUE ("event data")) -> (error out=w339:errorcluster)  [unwired: 2 in, 1 out]
            n114 = local read "Calling Mode"() -> (w359:T1)
            n115 = call-dynamic "Fire Quit Event.vi"("error in (no error)"=w339, "Force Quit?"=TRUE, "BaseSpecPage in"=w337) -> ("error out"=w338:errorcluster)  [unwired: 6 in, 2 out]
            n116 = local write "Error Messages"("") -> ()
            n117 = case shown="\"Open Recent Item\"" w359 {
              tunnel: [w361 w363 w365] -> w342
              frame Default {
                n118 = control-ref of="Back"() -> (w361:refnum<vi>)
                n119 = property on="Back" class="Bool"("Visible"=TRUE) -> ()  [unwired: 2 in, 2 out]
              }
              frame "Open Recent Item" {
                n120 = control-ref of="Next"() -> (w363:refnum<vi>)
                n121 = property on="Back" class="Bool"("Visible"=FALSE) -> ()  [unwired: 2 in, 2 out]
              }
              frame "Open to 2nd Page" {
                n122 = control-ref of="Next"() -> (w365:refnum<vi>)
              }
            }
            n123 = Bundle(cluster=w355, "\"Tab Forward To\" Refnum"=w342, "\"Tab Backward To\" Refnum"=w350, "Errors"=w354, "Quit"=w336) -> (w356:T7)
            n124 = call-by-ref "?"("error in (no error)"=w338, "Wizard Interface"=w356, "MetaDataObj"=w332) -> ("VI Ref Out"=w341:refnum<vi>, "BaseSpecPage out"=w340:refnum<class "BaseSpecPage.lvclass">, "SpecPage Ctrl #n Ref"=w357:refnum<vi>, "SpecPage Ctrl #1 Ref"=w358:refnum<vi>)  [unwired: 7 in, 2 out]
            n125 = local write "CurPage Ctrl #n"(w357) -> ()
            n126 = local write "CurPage Ctrl #1"(w358) -> ()
            n127 = control-ref of="Next"() -> ()  [unwired: 1 out]
            n128 = invoke class="VI" method="FP.Close"(reference=w341) -> (reference out=w360:refnum<vi>)  [unwired: 2 in, 2 out]
            n129 = Format Into String(format string="Spec Page Title", w331) -> (resulting string=w333:string)  [unwired: 2 in, 1 out]
            n130 = local write "Title"(w333) -> ()
            n131 = invoke on="Page Selector" class="SubPnl" method="Insert VI"("VI Ref"=w360) -> ()  [unwired: 3 in, 4 out]
            n132 = Equal?(x=w347, y=w344) -> (x = y?=w348:bool)
            n133 = property on="Error Messages" class="Str"("Visible"=TRUE) -> ()  [unwired: 2 in, 2 out]
            n134 = Select(t=w347, s=w348, f=T2."Standard" ("Front Panel Window:State")) -> (s? t:f=w345:T2)
          }
          frame #2 {
            n135 = control-ref of="This VI"() -> (w370:refnum<vi>)
            n136 = property class="VI"("FP.State"=w368) -> ()  [unwired: 2 in, 2 out]
            n137 = call-by-ref "?"("Defer?"=FALSE ("Visible"), "VI in"=w370) -> ()  [unwired: 11 in, 3 out]
          }
        }
      }
      frame "StopSpecPage" {
        # "Notify just the spec page to quit."
        n138 = call-dynamic "Fire Quit Event.vi"("error in (no error)"=w378, "BaseSpecPage in"=w380) -> ("error out"=w377:errorcluster, "Quit OK?"=w375:bool, "BaseSpecPage out"=w379:refnum<class "BaseSpecPage.lvclass">)  [unwired: 7 in]
        n139 = case shown="True" w375 {
          tunnel: [w392 w394] -> w386
          tunnel: [w391 refnum<class "BaseSpecPage.lvclass"> refnum ("BaseSpecPage out")] -> w381
          tunnel: w379 -> [w391 w397]
          tunnel: w377 -> [w388 w396]
          tunnel: [w387 w395] -> w376
          tunnel: w374 -> [w392 _]
          tunnel: w373 -> [w390 w393]
          tunnel: [w389 w393] -> w372
          frame False {
            n140 = Flush Queue(queue=w390, error in (no error)=w388) -> (queue out=w389:refnum<queue>, error out=w387:errorcluster)  [unwired: 1 out]
          }
          frame True {
            n141 = call-dynamic "Finalize.vi"("error in (no error)"=w396, "BaseSpecPage in"=w397) -> ("error out"=w395:errorcluster, "MetaDataObj out"=w394:refnum<class "MetaDataObj.lvclass">)  [unwired: 7 in, 1 out]
          }
        }
      }
      frame "Copy Project" {
        n142 = property class="MetaDataObj.lvclass"(reference=w416) -> (reference out=w411:refnum<class "MetaDataObj.lvclass">, "Project Path"=w419:path, "Project Root"=w415:path, "File Prefix"=w414:string, "Project Name"=w413:string, "Overlay Icon"=w412:refnum<class "Icon.lvclass">)  [unwired: 1 in, 1 out]
        n143 = Build Array(w415) -> (w420:path[])
        n144 = call-by-ref "?"("value"=w420, "key"=w406) -> ()  [unwired: 7 in, 3 out]
        n145 = call-by-ref "?"("File Path In"=w419) -> ("Valid File Path?"=w418:bool, "File Path Out"=w417:path)  [unwired: 11 in, 2 out]
        n146 = case shown="True" w418 {
          tunnel: w414 -> [_ w440]
          tunnel: w413 -> [_ w437]
          tunnel: w412 -> [_ w438]
          tunnel: w415 -> [_ w439]
          tunnel: w417 -> [_ w436]
          tunnel: w411 -> [_ w435]
          tunnel: w408 -> [w426 _]
          tunnel: [w426 w434] -> w407
          tunnel: w405 -> [w424 w431]
          tunnel: w404 -> [w425 w432]
          tunnel: [w423 w430] -> w403
          tunnel: [w422 w429] -> w402
          frame False {
            # "If the project source is not found, a dialog has already popped up...send Quit_Finish to close the Create Project dialog"
            n147 = One Button Dialog(message="File Not Found") -> ()  [unwired: 1 in, 1 out]
            n148 = Enqueue Element At Opposite End(queue=w425, element="Quit_Finish", error in (no error)=w424) -> (queue out=w423:refnum<queue>, error out=w422:errorcluster)  [unwired: 1 in, 1 out]
          }
          frame True {
            # "Set a busy cursor... this is the point of no return"
            n149 = call-by-ref "?"() -> ("error out"=w433:errorcluster)  [unwired: 12 in, 3 out]
            n150 = call-by-ref "?"("Overlay Icon"=w438, "Target Project Name"=w437, "MetaDataObj"=w435, "error in (no error)"=w433, "Target File Prefix"=w440, "Target Path"=w439, "Source Project Path"=w436) -> ("error out"=w428:errorcluster, "Project"=w434:refnum<vi>)  [unwired: 5 in, 2 out]
            n151 = case shown="Error" w428 {
              tunnel: w432 -> [w442 w446]
              tunnel: w431 -> [w441 w445]
              tunnel: [w442 w443] -> w430
              tunnel: [w441 w444] -> w429
              frame No Error {
              }
              frame Error {
                # "If an error happened during user project creation, an error dialog has already popped up...send Quit to close the Create Project dialog"
                n152 = Enqueue Element At Opposite End(queue=w446, element="Quit", error in (no error)=w445) -> (queue out=w443:refnum<queue>, error out=w444:errorcluster)  [unwired: 1 in, 1 out]
              }
            }
          }
        }
      }
      frame "Show Project" {
        # "Once the project window is shown, close its reference since it is now open\nand the NPW is about to close."
        n153 = flat-sequence {
          tunnel: w453 -> [w464]
          tunnel: [w463] -> w451
          frame #0 {
            n154 = property class="Project"(reference=w464) -> (reference out=w463:refnum<vi>, "Path"=w462:path)  [unwired: 1 in, 1 out]
            n155 = invoke class="App" method="Open.LV Document"("path"=w462) -> ()  [unwired: 4 in, 5 out]
          }
        }
        n156 = Enqueue Element(queue=w460, element="Quit", error in (no error)=w459) -> (queue out=w458:refnum<queue>, error out=w457:errorcluster)  [unwired: 1 in, 1 out]
        n157 = Close Reference(reference=w451) -> ()  [unwired: 1 in, 1 out]
      }
      frame "Quit" {
        # "Log selected project to CEIP."
        # "This is the first step of Quit, which should execute if the user did NOT cancel."
        n158 = call-by-ref "?"("Template"=w469) -> ()  [unwired: 13 in, 2 out]
        n159 = call-by-ref "?"("Operation to Log"=Operation_to_Log."Create", "MetaDataObj in"=w469) -> ()  [unwired: 12 in, 2 out]
        n160 = Enqueue Element At Opposite End(queue=w475, element="Quit_Finish", error in (no error)=w473) -> (queue out=w474:refnum<queue>, error out=w472:errorcluster)  [unwired: 1 in, 1 out]
      }
      frame "Quit_Finish" {
        # "This is the second phase of Quit, which should happen even if the user cancelled."
        # "Even though we don't need\nthe data, we wait so LV knows\nto release the record of this\nexecution."
        # "Notify both of the pages to quit."
        n161 = Obtain Queue(name (unnamed)="SearchPageQueue", element data type="", create if not found? (T)=FALSE) -> (queue out=w496:refnum<queue>, error out=w495:errorcluster)  [unwired: 2 in, 1 out]
        n162 = Enqueue Element(queue=w496, element="Quit", error in (no error)=w495) -> (queue out=w491:refnum<queue>, error out=w490:errorcluster)  [unwired: 1 in, 1 out]
        n163 = Release Queue(queue=w491, error in (no error)=w490) -> (error out=w483:errorcluster)  [unwired: 1 in, 2 out]
        n164 = call-dynamic "Fire Quit Event.vi"("error in (no error)"=w483, "Force Quit?"=TRUE, "BaseSpecPage in"=w478) -> ("error out"=w482:errorcluster, "BaseSpecPage out"=w481:refnum<class "BaseSpecPage.lvclass">)  [unwired: 6 in, 1 out]
        n165 = call-dynamic "Finalize.vi"("error in (no error)"=w482, "BaseSpecPage in"=w481) -> ("MetaDataObj out"=w480:refnum<class "MetaDataObj.lvclass">)  [unwired: 7 in, 2 out]
        n166 = flat-sequence {
          tunnel: w480 -> [_]
          frame #0 {
          }
        }
      }
    }
  }
  n167 = Close Reference(reference=w11) -> ()  [unwired: 1 in, 1 out]
  n168 = Unregister For Events(event registration refnum=w8, error in=w21) -> (error out=w5:errorcluster)
  n169 = Destroy User Event(user event=w35, error in=w5) -> (error out=w20:errorcluster)
  n170 = Destroy User Event(user event=w14, error in=w20) -> ()  [unwired: 1 out]
  n171 = case shown="False" w2 {
    tunnel: [w501 _] -> w1
    frame False {
      # "If not canceled, hide the panel, and give the plugin VI (either AfterPage1 or AfterPage2WithUI) a chance to show its panel before closing the NPW panel. This is to prevent the GSW from appearing in between these windows closing and opening."
      n172 = flat-sequence {
        tunnel: [errorcluster {"status"=FALSE, "code"=0, "source"=""} ("error constant")] -> w501
        frame #0 {
          n173 = property class="VI"("FP.State"=T2."Hidden" ("Front Panel Window:State")) -> ()  [unwired: 2 in, 2 out]
        }
        frame #1 {
          n174 = Wait (ms)(milliseconds to wait=u32 1000) -> ()  [unwired: 1 out]
        }
        frame #2 {
        }
      }
    }
    frame True {
    }
  }
  n175 = invoke class="VI" method="FP.Close"(error in=w1) -> ()  [unwired: 2 in, 3 out]
